vi "Convert Heading To Ship Rotation Texture Index.vi"(11 "Heading [deg]":sgl) -> (3 "Texture Index":i32)   [LabVIEW 2021, in "Ship.lvclass"]
uses:
  Ship.lvclass
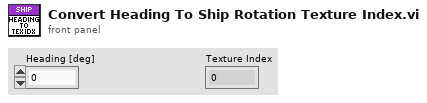
[diagram p1: front panel]
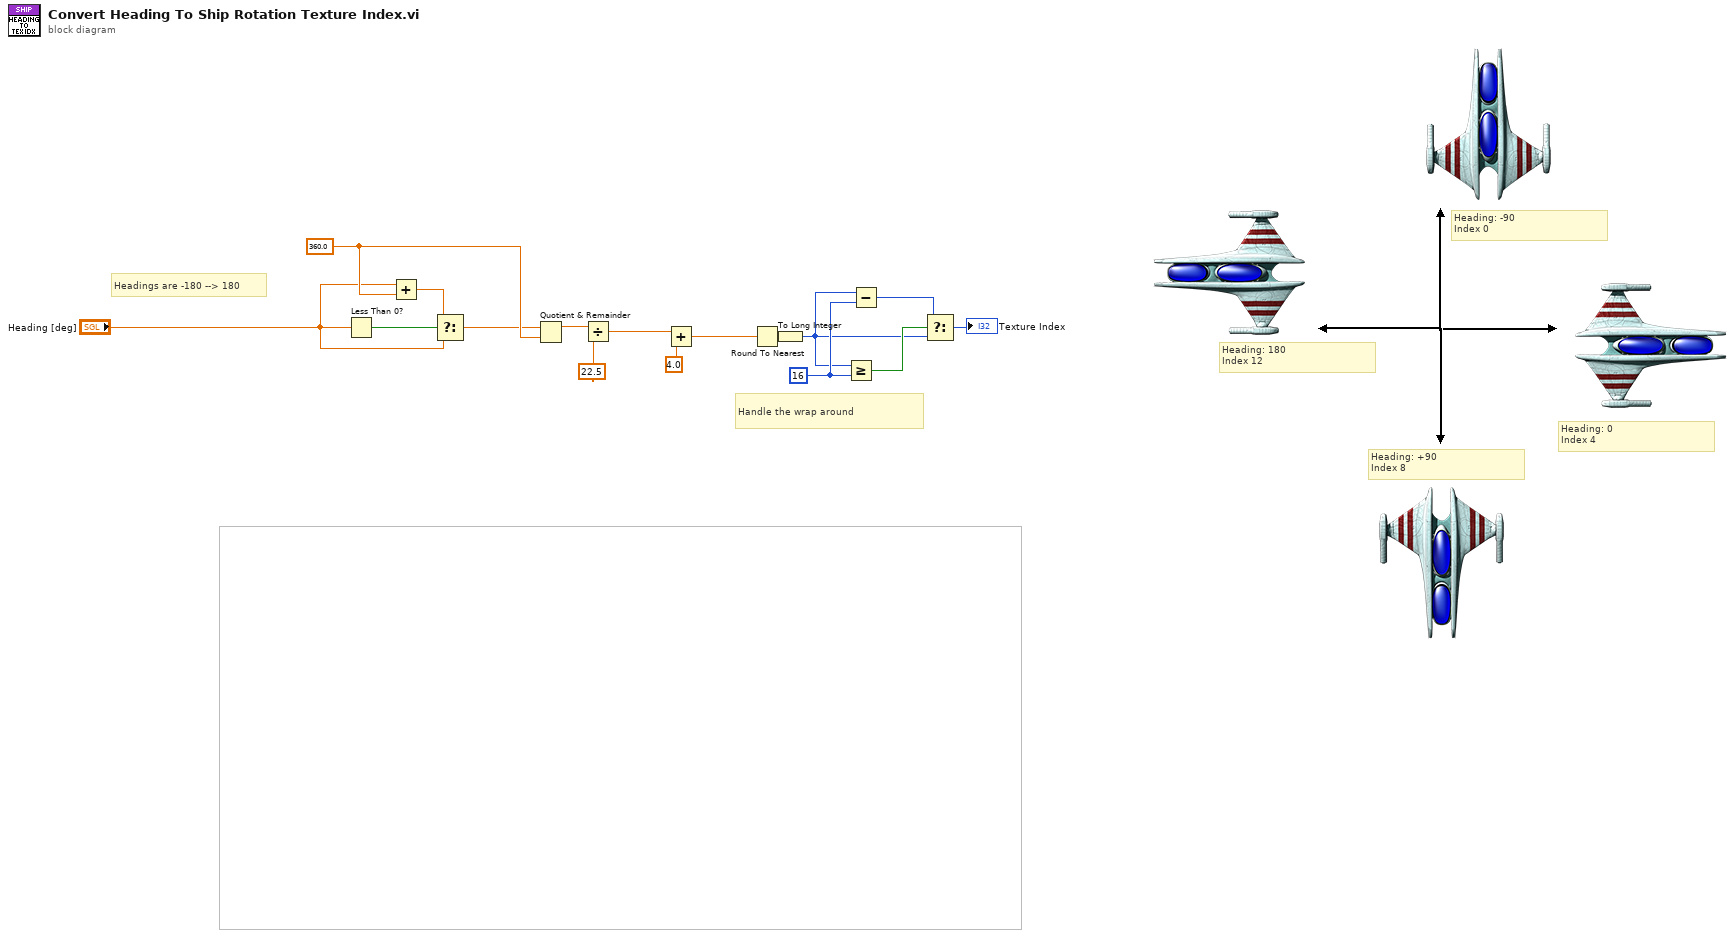
[diagram p0: block diagram]
diagram:
  w2 = 16 ("y")
  w14 = sgl 360.0 ("y")
  # "Headings are -180 --> 180"
  # "Handle the wrap around"
  # "Heading: -90\nIndex 0"
  # "Heading: 180\nIndex 12"
  # "Heading: +90\nIndex 8"
  # "Heading: 0\nIndex 4"
  n1 = Less Than 0?(x="Heading [deg]") -> (x < 0?=w16:bool)
  n2 = Add(x="Heading [deg]", y=w14) -> (x+y=w15:sgl)
  n3 = Select(t=w15, s=w16, f="Heading [deg]") -> (s? t:f=w13:sgl)
  n4 = Quotient & Remainder(x=w13, y=w14) -> (x-y*floor(x/y)=w9:sgl)  [unwired: 1 out]
  n5 = Divide(x=w9, y=sgl 22.5) -> (x/y=w10:sgl)
  n6 = Add(x=w10, y=sgl 4.0) -> (x+y=w5:sgl)
  n7 = Round To Nearest(number=w5) -> (nearest integer value=w3:sgl)
  n8 = To Long Integer(number=w3) -> (32bit integer=w1:i32)
  n9 = Greater Or Equal?(x=w1, y=w2) -> (x >= y?=w4:bool)
  n10 = Subtract(x=w1, y=w2) -> (x-y=w6:i32)
  n11 = Select(t=w6, s=w4, f=w1) -> (s? t:f=→"Texture Index":i32)
